vi "SetXL_CellValue_String.vi"(0 "Refnum Cluster In":T1, 5 "Start":cluster{"Column":i32, "Row":i32}, 7 "End":cluster{"Column":i32, "Row":i32}, 9 "data":string, 11 "error in (no error)":errorcluster) -> (4 "Refnum Cluster Out":T1, 15 "error out":errorcluster)   [LabVIEW 2017, in "excel_configuration.lvlib"]
doc: "Writes a string into a cell, or into the range between Start and End, of the open worksheet."
uses:
  excel_configuration.lvlib
  94c75aee-dd0c-4b76-843d-1cc6ea3be07d.vi
  <vilib>/Utility/error.llb/Clear Errors.vi
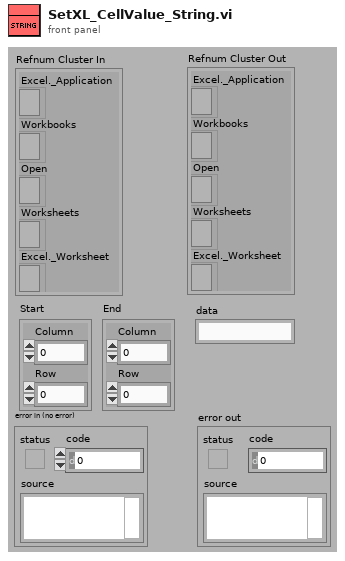
[diagram p1: front panel]
types:
  T1 = cluster{"Excel._Application":refnum<k7>, "Workbooks":refnum<k7>, "Open":refnum<k7>, "Worksheets":refnum<k7>, "Excel._Worksheet":refnum<k7>}
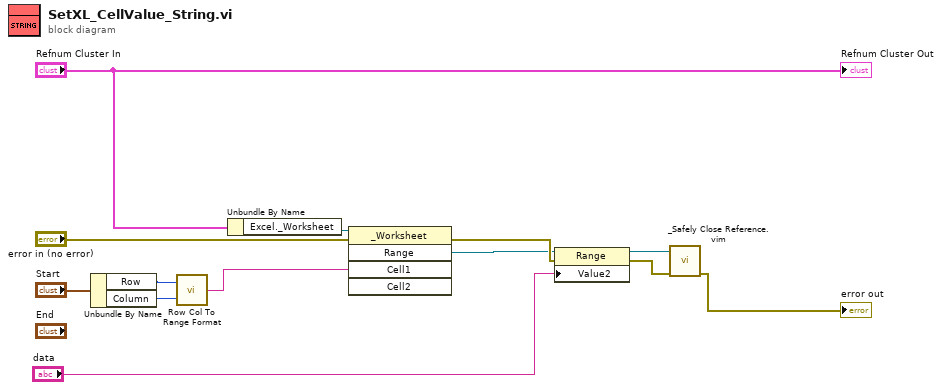
[diagram p0: block diagram]
diagram:
  n1 = Unbundle By Name("Start") -> ("Row"=w7:i32, "Column"=w6:i32)
  n2 = call "Row Col To Range Format.vi"("Column"=w6, "Row"=w7) -> ("Output String"=w5:string)
  n3 = Unbundle By Name("Refnum Cluster In") -> ("Excel._Worksheet"=w3:refnum<k7>)
  n4 = invoke class="_Worksheet" method="Range"(reference=w3, error in="error in (no error)", "Cell1"=w5) -> (error out=w12:errorcluster, "Range"=w11:refnum<k7>)  [unwired: 2 in, 3 out]
  n5 = property class="Range"(reference=w11, error in=w12, "Value2"="data") -> (reference out=w10:refnum<k7>, error out=w9:errorcluster)
  n6 = call "_Safely Close Reference.vim"("error in (no error)"=w9, "Automation Refnum in"=w10) -> ("error out"=→"error out":errorcluster)  [unwired: 9 in]
  "Refnum Cluster Out" <- "Refnum Cluster In"
